vi "Send IED Measurement Status.vi"(4 "Status":T1, 5 "IED Measurement Msg":refnum<class "IED Measurement Status Msg.lvclass">, 6 "Value/error":string, 7 "Message Priority (Normal)":T2=enum."Normal", 8 "error in (no error)":errorcluster, 9 "Measurement Name":string, 10 "IED Name":string, 11 "Message Enqueuer in":refnum<class "Message Enqueuer.lvclass">) -> (0 "error out":errorcluster, 3 "Message Enqueuer out":refnum<class "Message Enqueuer.lvclass">)   [LabVIEW 2015, in "SCADA Core.lvlib" / "IED Measurement Status Msg.lvclass"]
uses:
  IED Measurement Status Msg.lvclass
  <vilib>/ActorFramework/Message Enqueuer/Message Enqueuer.lvclass
  <vilib>/ActorFramework/Message Enqueuer/Message Priority.ctl
  IED Measurement Status.ctl
  IED Measurement Status Msg.lvclass/IED Measurement Status Msg.ctl
  <vilib>/ActorFramework/Message Enqueuer/Message Enqueuer.lvclass/Message Enqueuer.ctl
  <vilib>/ActorFramework/Message Priority Queue/Priority Enqueue.vi
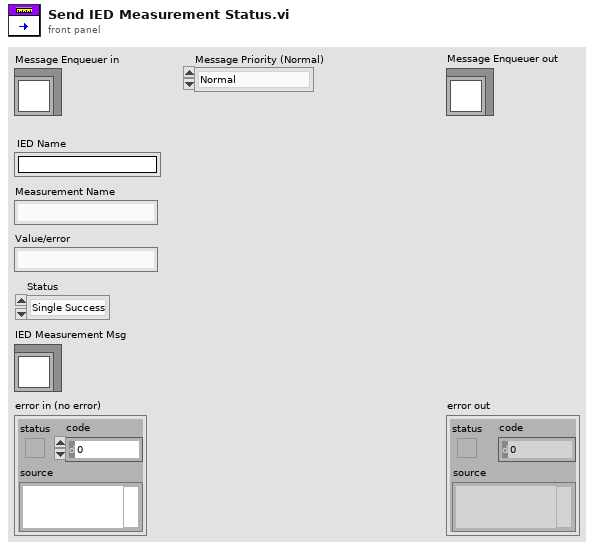
[diagram p1: front panel]
types:
  T1 = typedef "SCADA Core.lvlib/IED Measurement Status Msg.lvclass/IED Measurement Status.ctl" = enum16{"Single Success", "Single Failure", "Multiple Success", "Multiple Failure"}
  T2 = typedef "Actor Framework.lvlib/Message Enqueuer.lvclass/Message Priority.ctl" = enum16{"Low", "Normal", "High"}
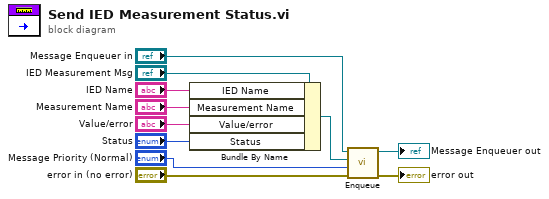
[diagram p0: block diagram]
diagram:
  n1 = Bundle By Name(cluster="IED Measurement Msg", "IED Name"="IED Name", "Measurement Name"="Measurement Name", "Value/error"="Value/error", "Status"="Status") -> (w10:refnum<class "IED Measurement Status Msg.lvclass">)
  n2 = call <vilib>:"Enqueue.vi"("error in (no error)"="error in (no error)", "Message Priority (Normal)"="Message Priority (Normal)", "Message"=w10, "Message Enqueuer in"="Message Enqueuer in") -> ("error out"=→"error out":errorcluster, "Message Enqueuer out"=→"Message Enqueuer out":refnum<class "Message Enqueuer.lvclass">)  [unwired: 6 in]
